vi "Chrg_Dschrg_new.vi"(0 "Data Task in":refnum<k21>, 1 "data task error in":errorcluster, 2 "#DAQ outputs (1-13)":i32, 4 "PS VISA in":refnum<visa-resource-name>, 5 "PS error in":errorcluster caption="NHR error in (no error)", 6 "DischargeCyclePath":path=path "C:/Users/ga11/Desktop/VI/results/3PtestCharge.lvm" caption="Filename", 7 "Charge/Discharge\n time":dbl, 8 "Charge/discharge":enum8{"Charge", "Discharge"}(ring), 9 "Charge/Discharge Voltage Setpoint":dbl format="%#.6g", 10 "CC or CCCV":enum16{"CC", "CCCV"}(ring), 11 "Current Setpoint":dbl format="%#.6g", 12 "Output Safety":T1, 13 "Current Cutoff":dbl) -> (14 "data task out":refnum<k21>, 15 "data task error out":errorcluster, 18 "PS VIS resource name out":refnum<visa-resource-name>, 19 "PS error out":errorcluster)   [LabVIEW 2020]
uses:
  Drivers-NHR-9200/NHR/NH Research Regenerative Test Series.lvlib
panel:
  out "WaitElapsed Time (s)":i32 caption="Elapsed Time (s)"
  out "PS error out 2":errorcluster
  out "error out":errorcluster
  out "Read Ave Current (A)":dbl
  out "Read Ave Voltage (V)":dbl
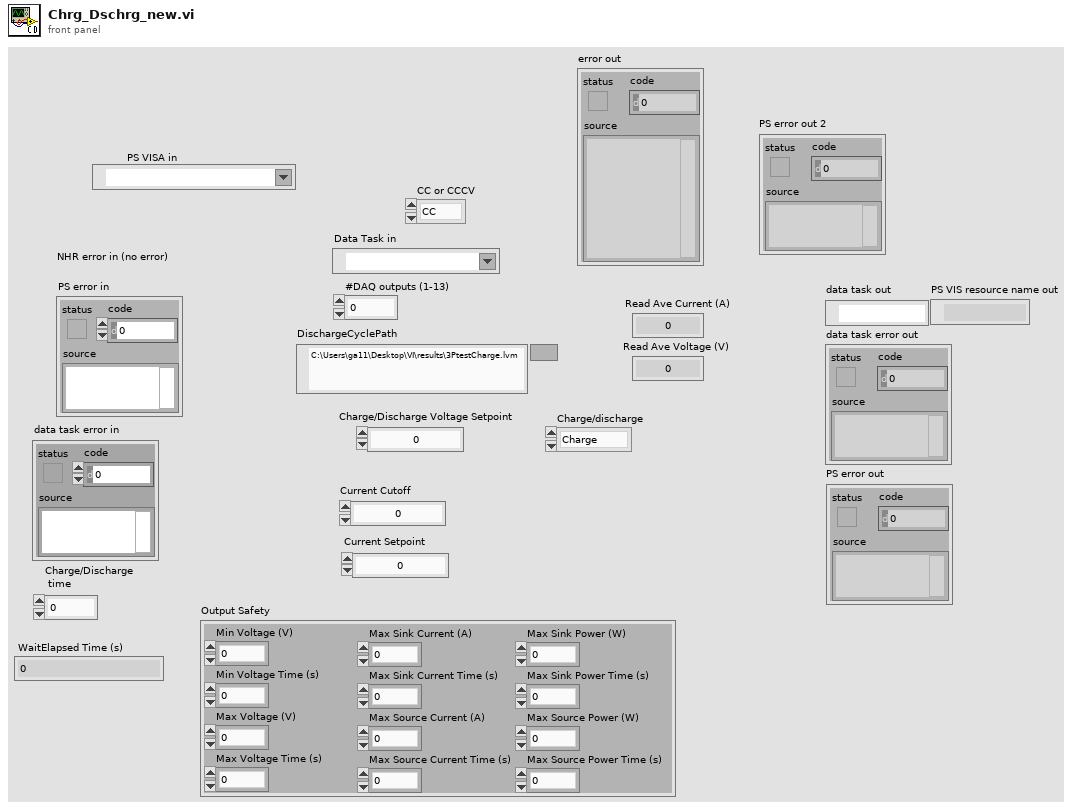
[diagram p1: front panel]
types:
  T1 = cluster{"Min Voltage (V)":dbl, "Min Voltage Time (s)":dbl, "Max Voltage (V)":dbl, "Max Voltage Time (s)":dbl, "Max Sink Current (A)":dbl, "Max Sink Current Time (s)":dbl, "Max Source Current (A)":dbl, "Max Source Current Time (s)":dbl, "Max Sink Power (W)":dbl, "Max Sink Power Time (s)":dbl, "Max Source Power (W)":dbl, "Max Source Power Time (s)":dbl}
  T2 = cluster{"Voltage Enabled":bool, "Current Enabled":bool, "Power Enabled":bool, "Resistance Enabled":bool}
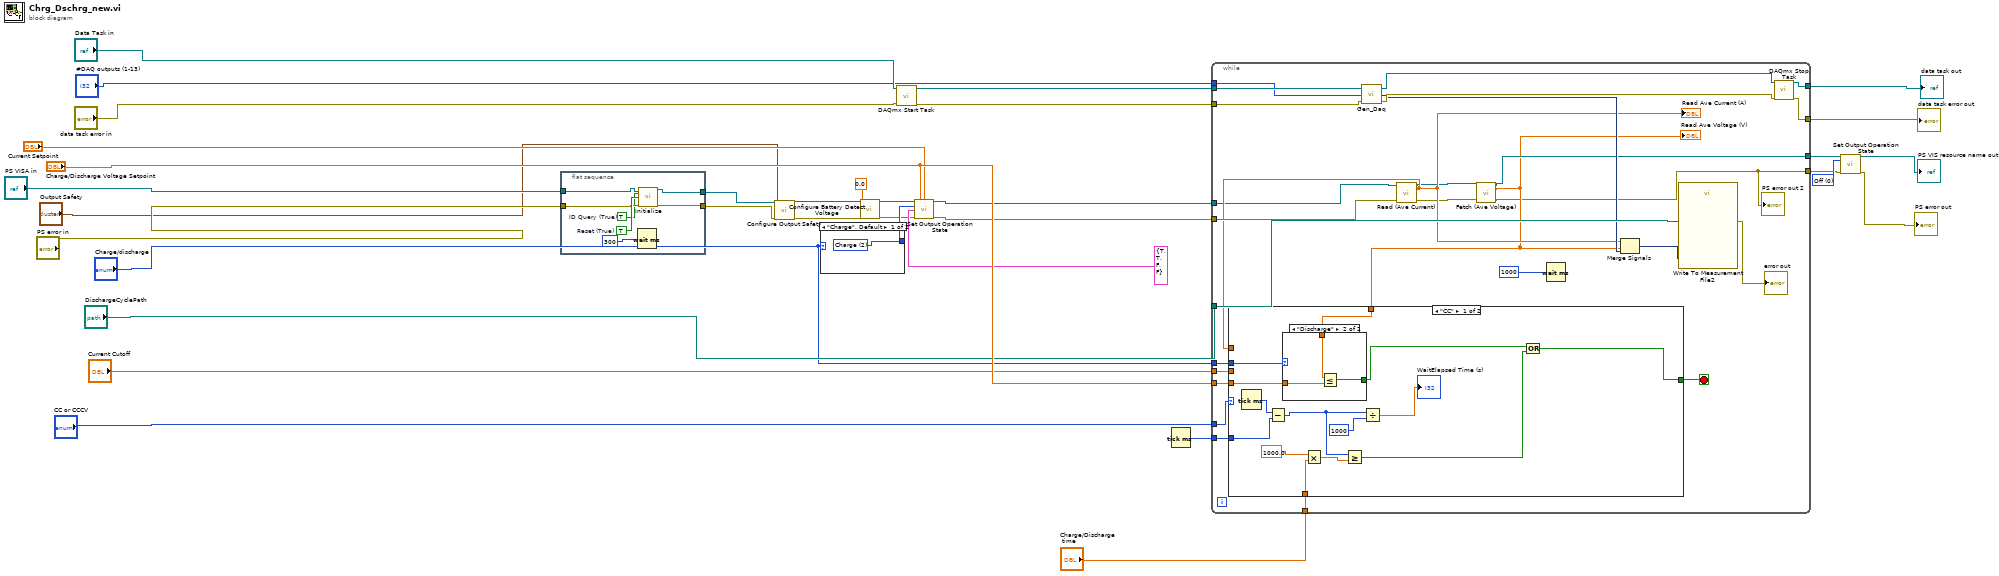
[diagram p0: block diagram]
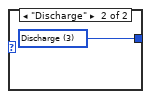
[diagram p2: hidden frame]
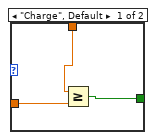
[diagram p3: hidden frame]
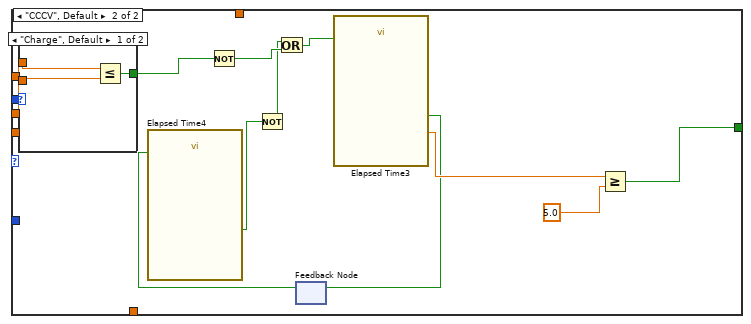
[diagram p4: hidden frame]
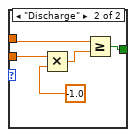
[diagram p5: hidden frame]
diagram:
  w12 = 0 items=["Off", "Standby", "Charge", "Discharge", "Battery"] ("Mode (0: Off)")
  n1 = flat-sequence {
    tunnel: [w36] -> w3
    tunnel: [w35] -> w4
    tunnel: "PS error in" -> [w38]
    tunnel: "PS VISA in" -> [w40]
    frame #0 {
      w39 = TRUE  # Reset (True)
      w37 = TRUE  # ID Query (True)
      n2 = Wait (ms)(milliseconds to wait=300) -> ()  [unwired: 1 out]
      n3 = call "Initialize.vi"("VISA resource name"=w40, "ID Query (True)"=w37, "Reset (True)"=w39, "error in (no error)"=w38) -> ("VISA resource name out"=w36:refnum<visa-resource-name>, "error out"=w35:errorcluster)  [unwired: 10 in]
    }
  }
  n4 = call "Configure Output Safety.vi"("VISA resource name"=w3, "Output Safety"="Output Safety", "error in (no error)"=w4) -> ("VISA resource name out"=w6:refnum<visa-resource-name>, "error out"=w5:errorcluster)  [unwired: 11 in]
  n5 = case shown="\"Charge\", Default" "Charge/discharge" {
    tunnel: [w42 w43] -> w15
    frame "Charge", Default {
      w42 = 2 items=["Off", "Standby", "Charge", "Discharge", "Battery"] ("Mode (0: Off)")
    }
    frame "Discharge" {
      w43 = 3 items=["Off", "Standby", "Charge", "Discharge", "Battery"] ("Mode (0: Off)")
    }
  }
  n6 = call "Configure Battery Detect Voltage.vi"("VISA resource name"=w6, "Battery Detect Voltage (0V)"=0.0, "error in (no error)"=w5) -> ("VISA resource name out"=w11:refnum<visa-resource-name>, "error out"=w10:errorcluster)  [unwired: 11 in]
  n7 = call <vilib>:"DAQmx Start Task.vi"("task/channels in"="Data Task in", "error in"="data task error in") -> ("task out"=w14:refnum<k21>, "error out"=w13:errorcluster)  [unwired: 12 in]
  n8 = call "Set Output Operation State.vi"("VISA resource name"=w11, "Voltage Setpoint (0 V)"="Charge/Discharge Voltage Setpoint", "Current Setpoint (0 A)"="Current Setpoint", "Mode (0: Off)"=w15, "Enable"=T2 {"Voltage Enabled"=TRUE, "Current Enabled"=TRUE, "Power Enabled"=FALSE, "Resistance Enabled"=FALSE}, "error in (no error)"=w10) -> ("VISA resource name out"=w18:refnum<visa-resource-name>, "error out"=w17:errorcluster)  [unwired: 8 in]
  n9 = Tick Count (ms)() -> (millisecond timer value=w2:u32)
  n10 = while {
    tunnel: w18 -> [w52]
    tunnel: w17 -> [w54]
    tunnel: "Current Cutoff" -> [w58]
    tunnel: w13 -> [w63]
    tunnel: w14 -> [w64]
    tunnel: "DischargeCyclePath" -> [w67]
    tunnel: [w66] -> w26
    tunnel: [w65] -> w24
    tunnel: [w49] -> w8
    tunnel: [w46] -> w7
    tunnel: "#DAQ outputs (1-13)" -> [w62]
    tunnel: "CC or CCCV" -> [w57]
    tunnel: "Charge/Discharge Voltage Setpoint" -> [w56]
    tunnel: "Charge/discharge" -> [w55]
    tunnel: w2 -> [w45]
    tunnel: "Charge/Discharge\n time" -> [w44]
    stop <- w68 stop-if-true
    n11 = call "Gen_Daq.vi"("error in"=w63, "#DAQ outputs (1-13)"=w62, "task/channels in"=w64) -> ("error out"=w60:errorcluster, "DaQ_output"=w59:dynamicdata, "task out"=w61:refnum<k21>)
    n12 = call "Read (Ave Current).vi"("VISA resource name"=w52, "error in (no error)"=w54) -> ("VISA resource name out"=w50:refnum<visa-resource-name>, "Ave Current (A)"=w53:dbl, "error out"=w51:errorcluster)  [unwired: 11 in]
    "Read Ave Current (A)" <- w53
    n13 = call "Fetch (Ave Voltage).vi"("VISA resource name"=w50, "error in (no error)"=w51) -> ("VISA resource name out"=w49:refnum<visa-resource-name>, "Ave Voltage (V)"=w48:dbl, "error out"=w46:errorcluster)  [unwired: 11 in]
    "Read Ave Voltage (V)" <- w48
    "PS error out 2" <- w46
    n14 = case shown="\"CC\"" w57 {
      tunnel: [w80 w97] -> w68
      tunnel: w58 -> [_ w94]
      tunnel: w53 -> [_ w93]
      tunnel: w48 -> [w83 _]
      tunnel: w56 -> [w84 _]
      tunnel: w55 -> [w82 w91]
      tunnel: w45 -> [w76 _]
      tunnel: w44 -> [w72 _]
      frame "CC" {
        n15 = Tick Count (ms)() -> (millisecond timer value=w77:u32)
        n16 = Subtract(x=w77, y=w76) -> (x-y=w73:u32)
        n17 = case shown="\"Discharge\"" w82 {
          tunnel: w84 -> [w86 w90]
          tunnel: w83 -> [w87 w89]
          tunnel: [w85 w88] -> w81
          frame "Charge", Default {
            n18 = Greater Or Equal?(x=w87, y=w86) -> (x >= y?=w85:bool)
          }
          frame "Discharge" {
            n19 = Less Or Equal?(x=w89, y=w90) -> (x <= y?=w88:bool)
          }
        }
        n20 = Multiply(x=1000.0, y=w72) -> (x*y=w75:dbl)
        n21 = Greater Or Equal?(x=w73, y=w75) -> (x >= y?=w71:bool)
        n22 = Divide(x=w73, y=1000) -> (x/y=→"WaitElapsed Time (s)":dbl)
        n23 = Or(x=w81, y=w71) -> (x .or. y?=w80:bool)
      }
      frame "CCCV", Default {
        n24 = case shown="\"Charge\", Default" w91 {
          tunnel: w94 -> [w105 w110]
          tunnel: w93 -> [w106 w108]
          tunnel: [w104 w107] -> w92
          frame "Charge", Default {
            n25 = Less Or Equal?(x=w106, y=w105) -> (x <= y?=w104:bool)
          }
          frame "Discharge" {
            n26 = Multiply(x=w110, y=-1.0) -> (x*y=w109:dbl)
            n27 = Greater Or Equal?(x=w108, y=w109) -> (x >= y?=w107:bool)
          }
        }
        n28 = Not(x=w92) -> (.not. x?=w103:bool)
        n29 = feedback #1() -> (w95:bool)  [unwired: 1 in]
        n30 = call "Elapsed Time4"("Reset"=w95) -> ("Time has Elapsed"=w102:bool)  [unwired: 11 in, 7 out]
        n31 = Not(x=w102) -> (.not. x?=w101:bool)
        n32 = Or(x=w101, y=w103) -> (x .or. y?=w100:bool)
        n33 = call "Elapsed Time3"("Reset"=w100) -> ("Elapsed Time (s)"=w99:dbl, "Time has Elapsed"=w96:bool)  [unwired: 11 in, 6 out]
        n34 = feedback-in #1(w96) -> ()
        n35 = Greater Or Equal?(x=w99, y=5.0) -> (x >= y?=w97:bool)
      }
    }
    n36 = Wait (ms)(milliseconds to wait=1000) -> ()  [unwired: 1 out]
    n37 = Merge Signals "Merge Signals"(w53, w48, w59) -> (w70:dynamicdata)
    n38 = call "Write To Measurement File2"("Signals"=w70, "Filename"=w67) -> ("error out"=→"error out":errorcluster)  [unwired: 15 in, 2 out]
    n39 = call <vilib>:"DAQmx Stop Task.vi"("task/channels in"=w61, "error in"=w60) -> ("task out"=w66:refnum<k21>, "error out"=w65:errorcluster)  [unwired: 12 in]
  }
  "data task out" <- w26
  "data task error out" <- w24
  n40 = call "Set Output Operation State.vi"("VISA resource name"=w8, "Mode (0: Off)"=w12, "error in (no error)"=w7) -> ("VISA resource name out"=→"PS VIS resource name out":refnum<visa-resource-name>, "error out"=→"PS error out":errorcluster)  [unwired: 11 in]
